vi "Release Agent.vi"(8 "error in (no error)":errorcluster, 11 "agent":T1) -> (0 "error out":errorcluster)   [LabVIEW 2013, in "libssh2.lvlib"]
uses:
  libssh2.lvlib
  Agent Refnum.ctl
  <vilib>/Utility/semaphor.llb/Release Semaphore.vi
  Read Session Refnum.vi
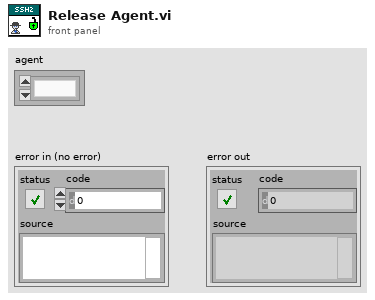
[diagram p1: front panel]
types:
  T1 = typedef "libssh2.lvlib/Agent Refnum.ctl" = refnum<k1>
  T2 = typedef "libssh2.lvlib/Session Refnum.ctl" = refnum<k1>
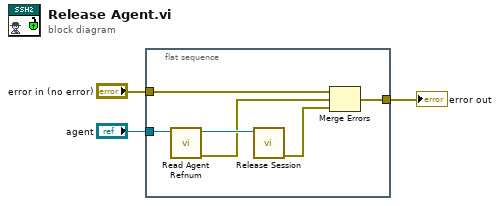
[diagram p0: block diagram]
diagram:
  n1 = flat-sequence {
    tunnel: [w6] -> w3
    tunnel: "error in (no error)" -> [w5]
    tunnel: "agent" -> [w4]
    frame #0 {
      n2 = call "Read Agent Refnum.vi"("agent"=w4) -> ("error out"=w8:errorcluster, "session"=w9:T2)  [unwired: 8 in, 1 out]
      n3 = call "Release Session.vi"("session"=w9) -> ("error out"=w7:errorcluster)  [unwired: 10 in]
      n4 = Merge Errors(w5, w8, w7) -> (w6:errorcluster)
    }
  }
  "error out" <- w3
